vi "ComPort.vi"() -> ()   [LabVIEW 2012]
uses:
  enum.ctl
panel:
  in  "file (use dialog)":path
  in  "Записать в файл":bool
  in  "6":bool
  in  "Stop":bool
  in  "5":bool
  in  "4":bool
  in  "3":bool
  in  "2":bool
  in  "1":bool
  in  "Tab Control":enum32{"A", "mA", "mkA", "F", "C", "Hz"}(tab)
  out "A":cluster{dbl[], dbl[]}[](graph)=[{array[625 elements], array[625 elements]}, {[46.166997484546506, 191.50003256887476, 217.56122335022303, 314.11051082895364, 367.6681204243802, 491.26342812001064, 547.3333894505861, 579.8709728432091, 610.6432728694004], [64.01945191125424, 63.99754492968501, 35.48635435349841, 18.605042994236122, 20.846827705685964, 8.006501966649115, 4.784517886488695, 5.45494186760662, 3.632449592605269]}]
  out "mA":cluster{dbl[], dbl[]}[](graph)=[{array[625 elements], array[625 elements]}, {[46.166997484546506, 191.50003256887476, 217.56122335022303, 314.11051082895364, 367.6681204243802, 491.26342812001064, 547.3333894505861, 579.8709728432091, 610.6432728694004], [64.01945191125424, 63.99754492968501, 35.48635435349841, 18.605042994236122, 20.846827705685964, 8.006501966649115, 4.784517886488695, 5.45494186760662, 3.632449592605269]}]
  out "mkA":cluster{dbl[], dbl[]}[](graph)=[{array[625 elements], array[625 elements]}, {[46.166997484546506, 191.50003256887476, 217.56122335022303, 314.11051082895364, 367.6681204243802, 491.26342812001064, 547.3333894505861, 579.8709728432091, 610.6432728694004], [64.01945191125424, 63.99754492968501, 35.48635435349841, 18.605042994236122, 20.846827705685964, 8.006501966649115, 4.784517886488695, 5.45494186760662, 3.632449592605269]}]
  out "F":cluster{dbl[], dbl[]}[](graph)=[{array[625 elements], array[625 elements]}, {[46.166997484546506, 191.50003256887476, 217.56122335022303, 314.11051082895364, 367.6681204243802, 491.26342812001064, 547.3333894505861, 579.8709728432091, 610.6432728694004], [64.01945191125424, 63.99754492968501, 35.48635435349841, 18.605042994236122, 20.846827705685964, 8.006501966649115, 4.784517886488695, 5.45494186760662, 3.632449592605269]}]
  out "C":cluster{dbl[], dbl[]}[](graph)=[{array[625 elements], array[625 elements]}, {[46.166997484546506, 191.50003256887476, 217.56122335022303, 314.11051082895364, 367.6681204243802, 491.26342812001064, 547.3333894505861, 579.8709728432091, 610.6432728694004], [64.01945191125424, 63.99754492968501, 35.48635435349841, 18.605042994236122, 20.846827705685964, 8.006501966649115, 4.784517886488695, 5.45494186760662, 3.632449592605269]}]
  out "Hz":cluster{dbl[], dbl[]}[](graph)=[{array[625 elements], array[625 elements]}, {[46.166997484546506, 191.50003256887476, 217.56122335022303, 314.11051082895364, 367.6681204243802, 491.26342812001064, 547.3333894505861, 579.8709728432091, 610.6432728694004], [64.01945191125424, 63.99754492968501, 35.48635435349841, 18.605042994236122, 20.846827705685964, 8.006501966649115, 4.784517886488695, 5.45494186760662, 3.632449592605269]}]
  out "Normal String":string
  out "Code string":string
  in  "parity":T1(ring)
  in  "stop bits":enum16{"1 bit", "1.5 bits", "2 bits"}(ring)
  in  "data bits":u16=8 min=5 max=8 step=1
  in  "baud rate":u32=9600
  in  "buffer size":u16
  in  "port number":i32
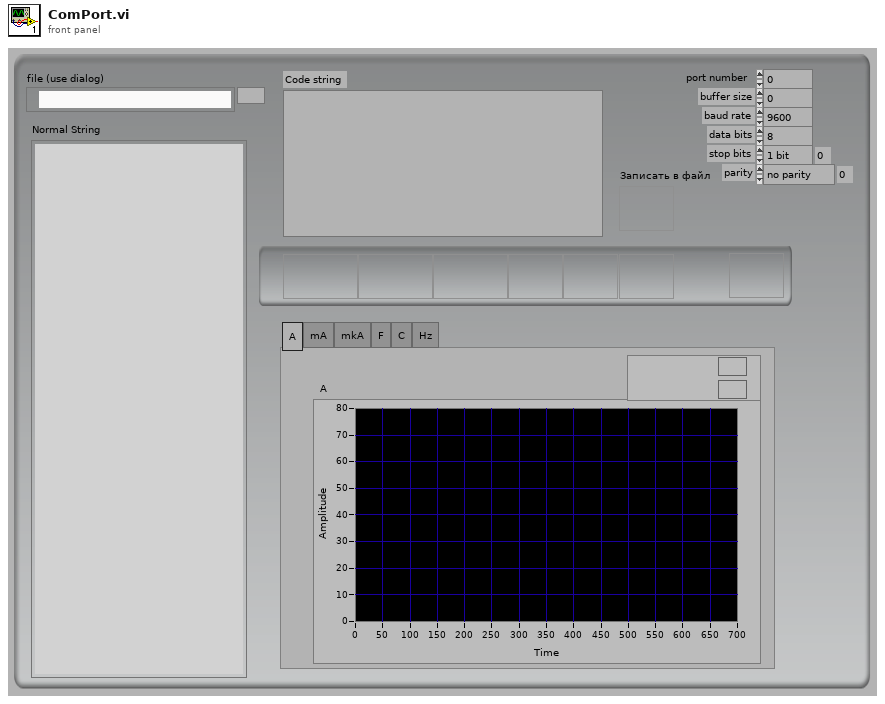
[diagram p1: front panel]
types:
  T1 = enum16{"no parity", "odd parity", "even parity", "mark parity", "space parity"}
  T2 = cluster{"baud rate":u32, "data bits":u16, "stop bits":enum16{"1 bit", "1.5 bits", "2 bits"}, "parity":enum16{"no parity", "odd parity", "even parity", "mark parity", "space parity"}, "buffer size":u16, "port number":i32, "Code String":string, "Normal String":string}
  T3 = typedef "enum.ctl" = enum16{"Initialize", "Duplicate case", "Close Serial Driver", "Serial Port Init", "Serial Line ctrl", "Serial Port Read", "V string", "Change parameters", "Write to txt file", "Stop"}
  T4 = cluster{"baud rate":u32, "data bits":u16, "stop bits":enum16{"1 bit", "1.5 bits", "2 bits"}, "parity":enum16{"no parity", "odd parity", "even parity", "mark parity", "space parity"}, "buffer size":u16, "port number":i32}
  T5 = enum16{"noop", "clear DTR", "set DTR", "clear RTS", "set RTS", "set DTR protocol", "clr DTR protocol", "noop2"}
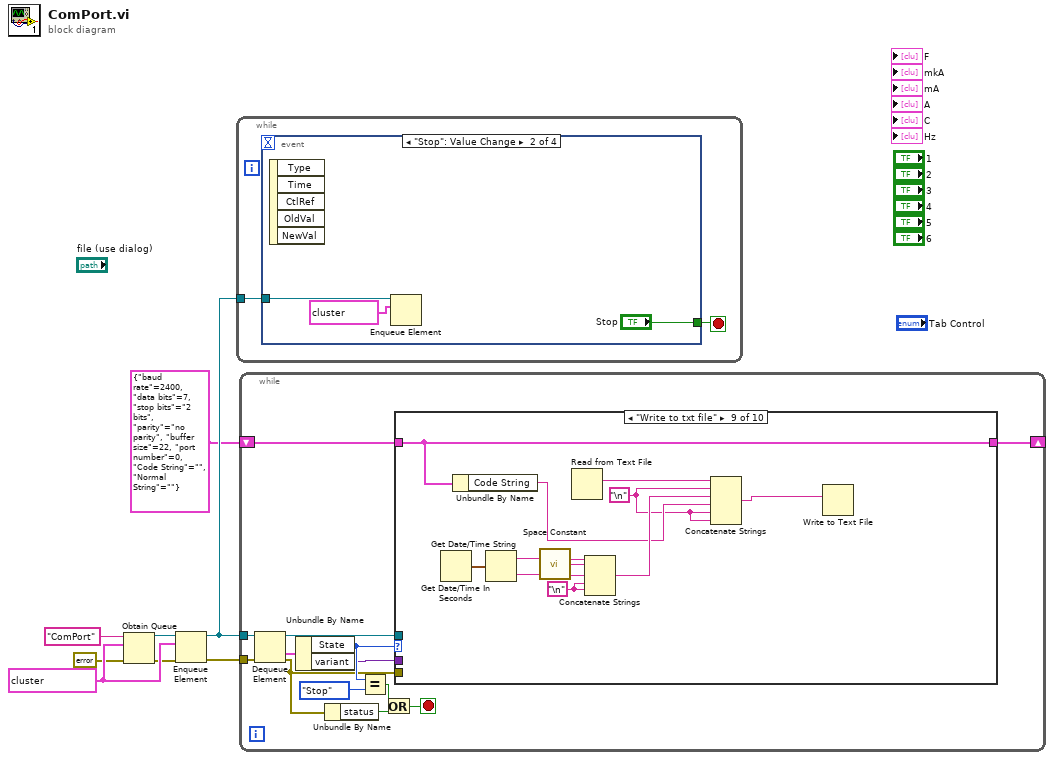
[diagram p0: block diagram]
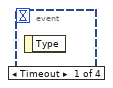
[diagram p2: hidden frame]
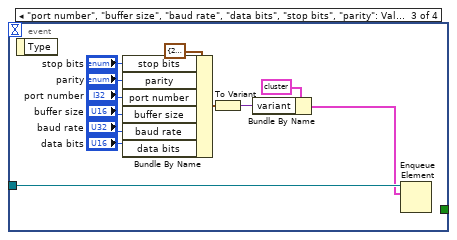
[diagram p3: hidden frame]
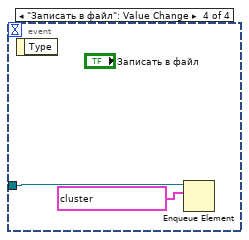
[diagram p4: hidden frame]
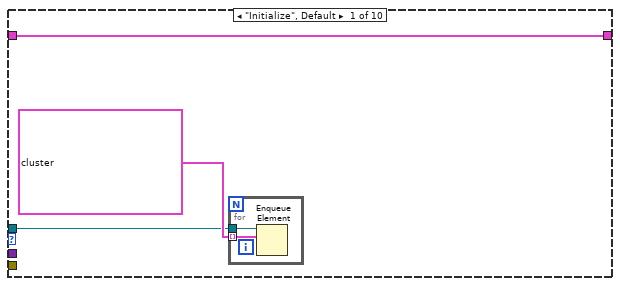
[diagram p5: hidden frame]
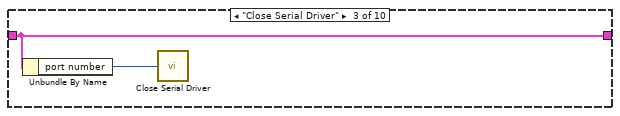
[diagram p7: hidden frame]
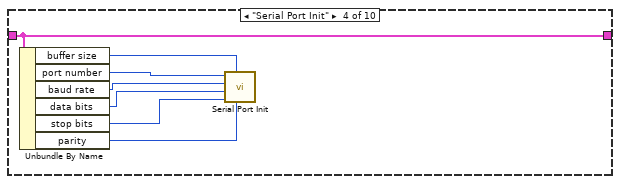
[diagram p8: hidden frame]
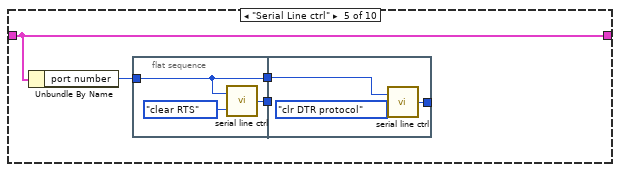
[diagram p9: hidden frame]
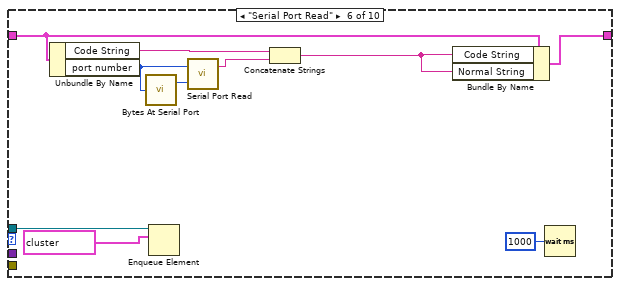
[diagram p10: hidden frame]
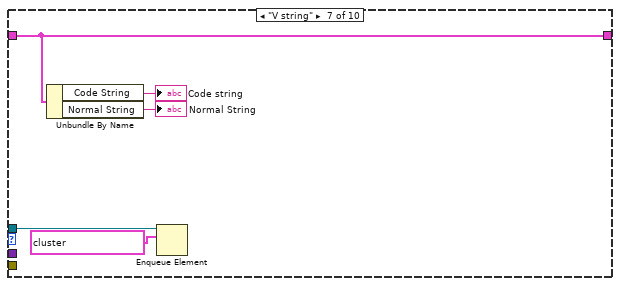
[diagram p11: hidden frame]
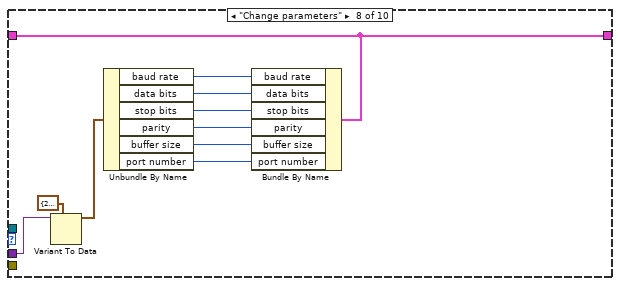
[diagram p12: hidden frame]
diagram:
  w6 = cluster{"variant":variant, "State":T3} {"variant"=variant, "State"=enum."Initialize"}
  n1 = Obtain Queue(name (unnamed)="ComPort", element data type=w6, error in (no error)=errorcluster {"status"=FALSE, "code"=0, "source"=""}) -> (queue out=w7:refnum<queue>, error out=w4:errorcluster)  [unwired: 2 in, 1 out]
  n2 = Enqueue Element(queue=w7, element=w6, error in (no error)=w4) -> (queue out=w5:refnum<queue>, error out=w2:errorcluster)  [unwired: 1 in, 1 out]
  n3 = while {
    tunnel: w5 -> [w10]
    stop <- w9 stop-if-true
    n4 = event shown="[1] \"Stop\": Value Change" {
      selector: _ -> [_ _ _ _]
      dyn-events: _ -> [_ _ _ _]
      timeout: _ -> [_ _ _ _]
      tunnel: w10 -> [_ w12 w18 w26]
      tunnel: [_ "Stop" _ _] -> w9
      event Timeout {
        n5 = event-data() -> ()  [unwired: 1 in, 1 out]
      }
      event "Stop": Value Change {
        n6 = event-data() -> ()  [unwired: 1 in, 5 out]
        n7 = Enqueue Element(queue=w12, element=cluster{"variant":variant, "State":T3} {"variant"=variant, "State"=enum."Stop"}) -> ()  [unwired: 2 in, 3 out]
      }
      event "port number", "buffer size", "baud rate", "data bits", "stop bits", "parity": Value Change {
        n8 = event-data() -> ()  [unwired: 1 in, 1 out]
        n9 = Bundle By Name(cluster=T4 {"baud rate"=2400, "data bits"=7, "stop bits"=enum."2 bits", "parity"=enum."no parity", "buffer size"=22, "port number"=0}, "stop bits"="stop bits", "parity"="parity", "port number"="port number", "buffer size"="buffer size", "baud rate"="baud rate", "data bits"="data bits") -> (w16:T4)
        n10 = To Variant(anything=w16) -> (Variant=w15:variant)
        n11 = Bundle By Name(cluster=cluster{"variant":variant, "State":T3} {"variant"=variant, "State"=enum."Change parameters"}, "variant"=w15) -> (w14:cluster{"variant":variant, "State":T3})
        n12 = Enqueue Element(queue=w18, element=w14) -> ()  [unwired: 2 in, 3 out]
      }
      event "Записать в файл": Value Change {
        n13 = event-data() -> ()  [unwired: 1 in, 1 out]
        n14 = Enqueue Element(queue=w26, element=cluster{"variant":variant, "State":T3} {"variant"=variant, "State"=enum."Write to txt file"}) -> ()  [unwired: 2 in, 3 out]
      }
    }
  }
  n15 = while {
    tunnel: w5 -> [w40]
    tunnel: w2 -> [w35]
    shift-right: [w29] -> _
    shift-left: T2 {"baud rate"=2400, "data bits"=7, "stop bits"=enum."2 bits", "parity"=enum."no parity", "buffer size"=22, "port number"=0, "Code String"="", "Normal String"=""} -> [w30]
    stop <- w32 stop-if-true
    n16 = Dequeue Element(queue=w40, error in (no error)=w35) -> (queue out=w39:refnum<queue>, element=w38:cluster{"variant":variant, "State":T3}, error out=w31:errorcluster)  [unwired: 1 in, 1 out]
    n17 = Unbundle By Name(w38) -> ("State"=w37:T3, "variant"=w28:variant)
    n18 = Unbundle By Name(w31) -> ("status"=w34:bool)
    n19 = Equal?(x=w37, y=enum."Stop" ("State")) -> (x = y?=w33:bool)
    n20 = Or(x=w33, y=w34) -> (x .or. y?=w32:bool)
    n21 = case shown="\"Write to txt file\"" w37 {
      tunnel: w39 -> [w41 _ _ _ _ w72 w76 _ _ _]
      tunnel: w31 -> [_ _ _ _ _ _ _ _ _ _]
      tunnel: w30 -> [w43 w46 w47 w55 w59 w70 w78 w88 w101 w102]
      tunnel: [w43 w46 w47 w55 w59 w69 w78 w88 w101 w102] -> w29
      tunnel: w28 -> [_ _ _ _ _ _ _ w90 _ _]
      frame "Initialize", Default {
        n22 = for {
          tunnel: w41 -> [w45]
          tunnel: cluster{"variant":variant, "State":T3}[] [{"variant"=variant, "State"=enum."Close Serial Driver"}, {"variant"=variant, "State"=enum."Serial Port Init"}, {"variant"=variant, "State"=enum."Serial Line ctrl"}, {"variant"=variant, "State"=enum."Serial Port Read"}] -> [w44] mode=indexing
          n23 = Enqueue Element(queue=w45, element=w44) -> ()  [unwired: 2 in, 3 out]
        }
      }
      frame "Duplicate case" {
      }
      frame "Close Serial Driver" {
        n24 = Unbundle By Name(w47) -> ("port number"=w48:i32)
        n25 = call <vilib>:"Close Serial Driver.vi"("port number"=w48) -> ()  [unwired: 1 out]
      }
      frame "Serial Port Init" {
        n26 = Unbundle By Name(w55) -> ("buffer size"=w54:u16, "port number"=w53:i32, "baud rate"=w52:u32, "data bits"=w51:u16, "stop bits"=w50:enum16{"1 bit", "1.5 bits", "2 bits"}, "parity"=w49:T1)
        n27 = call <vilib>:"Serial Port Init.vi"("parity"=w49, "buffer size"=w54, "stop bits"=w50, "data bits"=w51, "baud rate"=w52, "port number"=w53) -> ()  [unwired: 1 in, 1 out]
      }
      frame "Serial Line ctrl" {
        n28 = Unbundle By Name(w59) -> ("port number"=w56:i32)
        n29 = flat-sequence {
          tunnel: [w61] -> w58
          tunnel: [w60] -> w57
          tunnel: w56 -> [w60]
          tunnel: w58 -> [_]
          tunnel: [w64] -> _
          tunnel: w57 -> [w63]
          frame #0 {
            n30 = call <vilib>:"serial line ctrl.vi"("function"=T5."clear RTS", "port number"=w60) -> ("error code"=w61:i32)
          }
          frame #1 {
            n31 = call <vilib>:"serial line ctrl.vi"("function"=T5."clr DTR protocol", "port number"=w63) -> ("error code"=w64:i32)
          }
        }
      }
      frame "Serial Port Read" {
        n32 = Unbundle By Name(w70) -> ("Code String"=w68:string, "port number"=w73:i32)
        n33 = call <vilib>:"Bytes At Serial Port.vi"("port number"=w73) -> ("byte count"=w75:u32)  [unwired: 1 out]
        n34 = Enqueue Element(queue=w72, element=cluster{"variant":variant, "State":T3} {"variant"=variant, "State"=enum."V string"}) -> ()  [unwired: 2 in, 3 out]
        n35 = call <vilib>:"Serial Port Read.vi"("requested byte count"=w75, "port number"=w73) -> ("string read"=w67:string)  [unwired: 1 out]
        n36 = Concatenate Strings(w68, w67) -> (w66:string)
        n37 = Bundle By Name(cluster=w70, "Code String"=w66, "Normal String"=w66) -> (w69:T2)
        n38 = Wait (ms)(milliseconds to wait=u32 1000) -> ()  [unwired: 1 out]
      }
      frame "V string" {
        n39 = Unbundle By Name(w78) -> ("Code String"=→"Code string":string, "Normal String"=→"Normal String":string)
        n40 = Enqueue Element(queue=w76, element=cluster{"variant":variant, "State":T3} {"variant"=variant, "State"=enum."Serial Port Read"}) -> ()  [unwired: 2 in, 3 out]
      }
      frame "Change parameters" {
        n41 = Variant To Data(type=T4 {"baud rate"=2400, "data bits"=7, "stop bits"=enum."2 bits", "parity"=enum."no parity", "buffer size"=22, "port number"=0}, Variant=w90) -> (data=w87:T4)  [unwired: 1 in, 1 out]
        n42 = Unbundle By Name(w87) -> ("baud rate"=w86:u32, "data bits"=w85:u16, "stop bits"=w84:enum16{"1 bit", "1.5 bits", "2 bits"}, "parity"=w83:T1, "buffer size"=w82:u16, "port number"=w81:i32)
        n43 = Bundle By Name(cluster=w88, "baud rate"=w86, "data bits"=w85, "stop bits"=w84, "parity"=w83, "buffer size"=w82, "port number"=w81) -> ()  [unwired: 1 out]
      }
      frame "Write to txt file" {
        w91 = "\n"
        w92 = "\n"
        n44 = Get Date/Time In Seconds() -> (seconds since 1Jan1904=w99:timestamp)
        n45 = Unbundle By Name(w101) -> ("Code String"=w93:string)
        n46 = Get Date/Time String(seconds (now)=w99) -> (date string=w97:string, time string=w95:string)  [unwired: 2 in]
        n47 = call <vilib>:"Space Constant.vi"() -> ("String"=w96:string)
        n48 = Read from Text File() -> (text=w100:string)  [unwired: 4 in, 3 out]
        n49 = Concatenate Strings(w97, w96, w95, w91, w91) -> (w94:string)
        n50 = Concatenate Strings(w100, w92, w94, w93, w92, w92) -> (w98:string)
        n51 = Write to Text File(text=w98) -> ()  [unwired: 3 in, 3 out]
      }
      frame "Stop" {
      }
    }
  }
